vi "OE_report_generation.vi"(8 "error in (no error)":errorcluster, 11 "Column Header and data":string[][](array[string])) -> (0 "error out":errorcluster)   [LabVIEW 2017]
uses:
  <vilib>/Utility/file.llb/Write Delimited Spreadsheet (string).vi
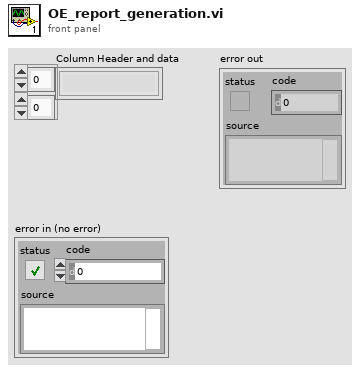
[diagram p1: front panel]
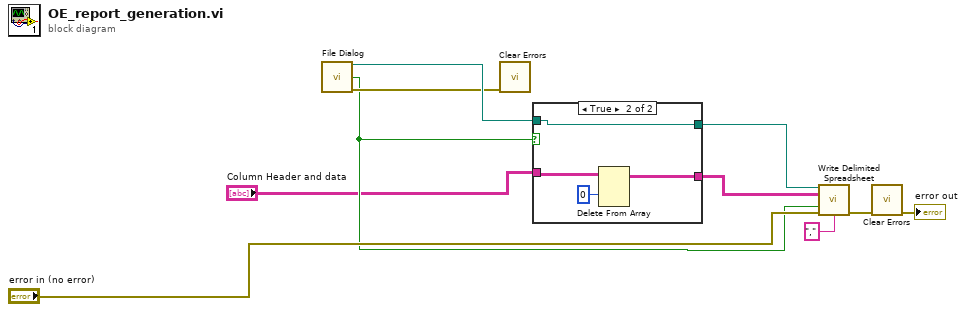
[diagram p0: block diagram]
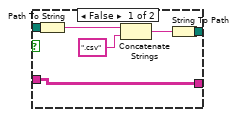
[diagram p2: hidden frame]
diagram:
  n1 = call "File Dialog"() -> ("selected path"=w7:path, "exists"=w3:bool, "error out"=w6:errorcluster)  [unwired: 12 in, 1 out]
  n2 = call <vilib>:"Clear Errors.vi"("error in (no error)"=w6) -> ()  [unwired: 5 in, 2 out]
  n3 = case shown="True" w3 {
    tunnel: [w16 w20] -> w8
    tunnel: w7 -> [w13 w20]
    tunnel: "Column Header and data" -> [w11 w19]
    tunnel: [w11 w17] -> w1
    frame False {
      n4 = Path To String(path=w13) -> (string=w14:string)
      n5 = Concatenate Strings(w14, ".csv" ("string")) -> (w15:string)
      n6 = String To Path(string=w15) -> (path=w16:path)
    }
    frame True {
      n7 = Delete From Array(array=w19, index (row)=0) -> (array with subset deleted=w17:string[][])  [unwired: 2 in, 1 out]
    }
  }
  n8 = call-poly <vilib>:"Write Delimited Spreadsheet.vi"("file path (dialog if empty)"=w8, "2D data"=w1, "append to file? (new file:F)"=w3, "error in (no error)"="error in (no error)", "delimiter (\\t)"="," ("delimiter (\\t)")) -> ("error out"=w4:errorcluster)  [unwired: 9 in, 1 out]
  n9 = call <vilib>:"Clear Errors.vi"("error in (no error)"=w4) -> ("error out"=→"error out":errorcluster)  [unwired: 5 in, 1 out]
